vi "UART Init.vi"(4 "TX GPIO":T1=16, 5 "Term Char (None)":string, 6 "RX GPIO":T1=17, 7 "UART #":T2, 8 "error in (no error)":errorcluster, 10 "Baud":u32=115200, 11 "DeviceComms in":refnum<class "DeviceComms.lvclass">) -> (0 "error out":errorcluster, 3 "DeviceComms out":refnum<class "DeviceComms.lvclass">)   [LabVIEW 2020, in "CTI.lvlib" / "DeviceComms.lvclass"]
uses:
  DeviceComms.lvclass
  UART Number.ctl
  CTI.lvlib
  GPIO Number.ctl
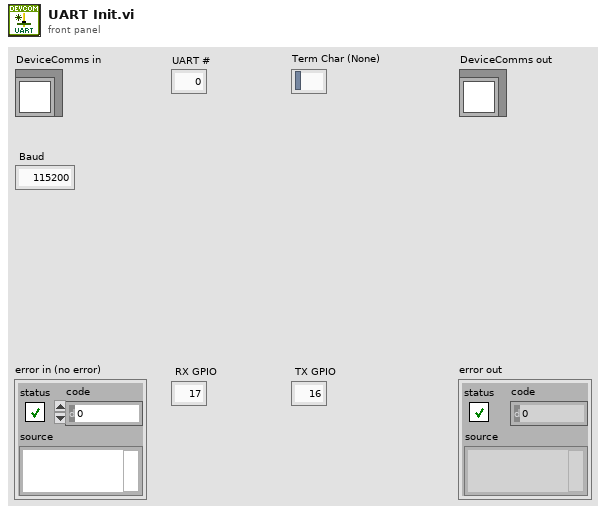
[diagram p1: front panel]
types:
  T1 = typedef "CTI.lvlib/GPIO Number.ctl" = i8
  T2 = typedef "CTI.lvlib/UART Number.ctl" = i8
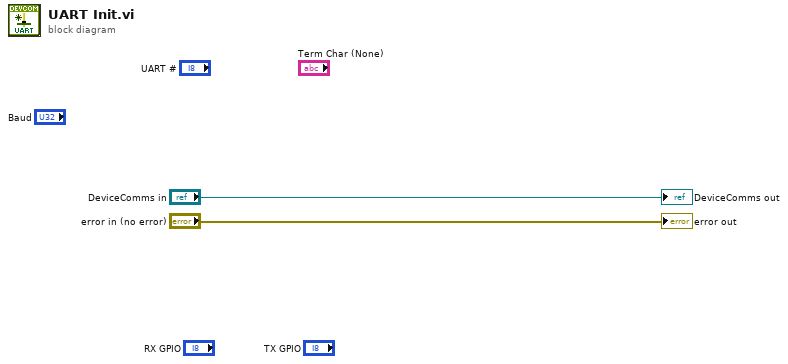
[diagram p0: block diagram]
diagram:
  "error out" <- "error in (no error)"
  "DeviceComms out" <- "DeviceComms in"
